vi "Update Monitor.Values by ID.vi"(8 "error in":errorcluster, 11 "Data":T1) -> (0 "error out":errorcluster)   [LabVIEW 2021, in "XNET-CAN-Signal-Logger.lvlib"]
uses:
  XNET-CAN-Signal-Logger.lvlib
  Typedef/Def-Data Queue Type.ctl
  Global Variables.vi
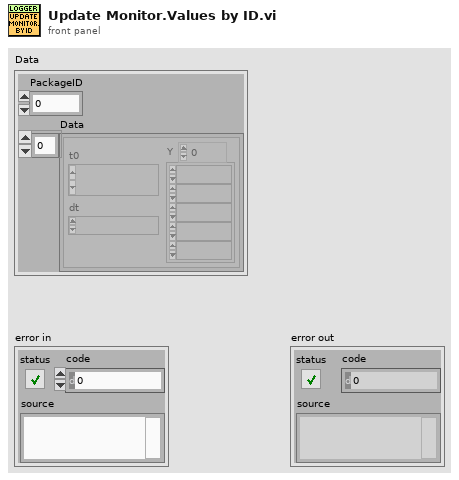
[diagram p1: front panel]
types:
  T1 = typedef "XNET-CAN-Signal-Logger.lvlib/Def-Data Queue Type.ctl" = cluster{"PackageID":i32, "Data":waveform(dbl)[]}
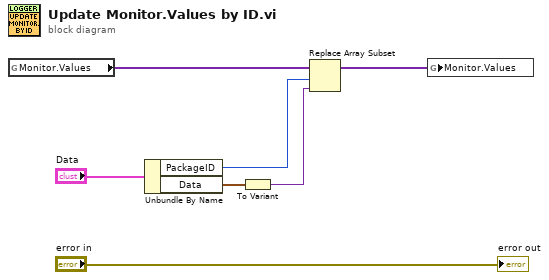
[diagram p0: block diagram]
diagram:
  n1 = global read "Global Variables.vi" "Monitor.Values"() -> (w7:variant[])
  n2 = Unbundle By Name("Data") -> ("PackageID"=w3:i32, "Data"=w2:waveform(dbl)[])
  n3 = To Variant(anything=w2) -> (Variant=w1:variant)
  n4 = Replace Array Subset(array=w7, new element=w1, index=w3) -> (w5:variant[])
  n5 = global write "Global Variables.vi" "Monitor.Values"(w5) -> ()
  "error out" <- "error in"
